vi "Measure Pulsed MinMax Mode.vi"(0 "Current level (A)":dbl=1e-06 format="%_4e", 1 "Current Source Reference In":string="6221", 2 "Voltage Source Reference In":refnum<visa-resource-name>="GPIB0::7::INSTR", 5 "Current Source Range":dbl=1e-05 step=1.0 format="%.4e", 7 "Current Pulse Frequency":dbl=2.0 format="%.4f", 9 "Current Source Compliance (V)":dbl=10.0 min=0.1 max=105.0 step=1.0 format="%.2e", 11 "Averaging time (s)":dbl=20.0, 12 "Voltmeter Wait (ms)":u32=900, 13 "Voltage Buffer Size":i32=60, 14 "Voltmeter Integration (NPLC)":dbl=1.0) -> (4 "Current Source Reference Out":string="6221", 6 "Voltmeter Reference Out":refnum<visa-resource-name>="GPIB0::7::INSTR", 8 "Resistance":dbl=1.1159355882352944, 10 "Error Out Current Source":errorcluster, 15 "Error Out Voltmeter":errorcluster)   [LabVIEW 2020]
uses:
  <vilib>/Analysis/baseanly.llb/Mean (DBL).vi
  <instrlib>/Keithley 2182/Keithley 2182.lvlib
  <vilib>/Analysis/NI_AALBase.lvlib
panel:
  out "i":i32=17
  out "Max-Min (V)":dbl=2.13487e-06
  out "Waveform Chart":dbl(graph)=1.0674350000000001
  in  "Current Pulse Offset":dbl format="%.4e"
  in  "phase mark channel":i32(ring)=1003 items=["TLINK 1"=1001, "TLINK 2"=1002, "TLINK 3"=1003, "TLINK 4"=1004, "None"=-1]
  in  "duty cycle":dbl=50.0 min=0.0 max=100.0 step=10.0 format="%.4f"
  in  "phase mark degrees":dbl=180.0 min=-180.0 max=180.0 step=15.0 format="%.4f"
  in  "Waveform":i32(ring)=2 items=["Sine"=1, "Square"=2, "Triangle"=3, "Ramp Up"=4, "Ramp Down"=5, "DC"=6]
  in  "Error In Voltage source":errorcluster
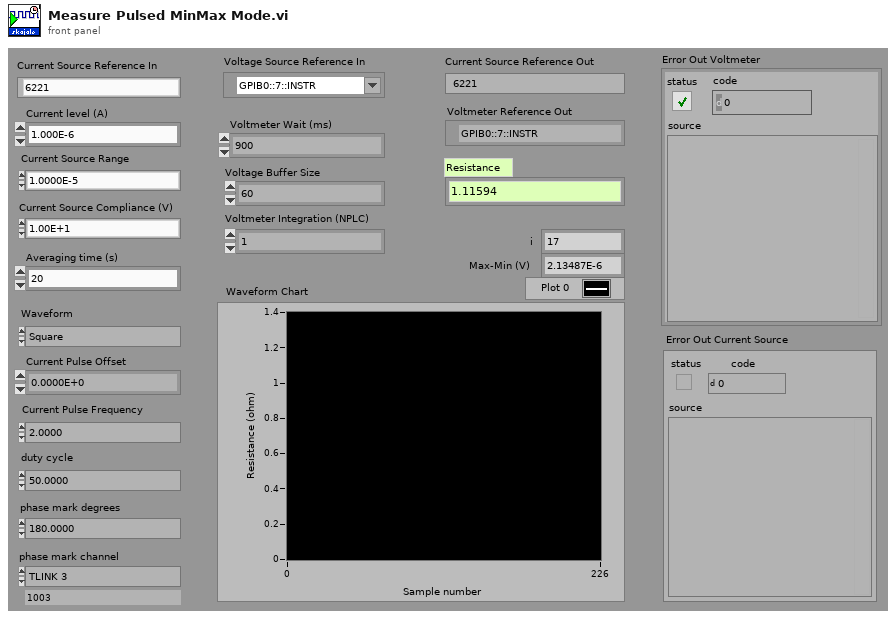
[diagram p1: front panel]
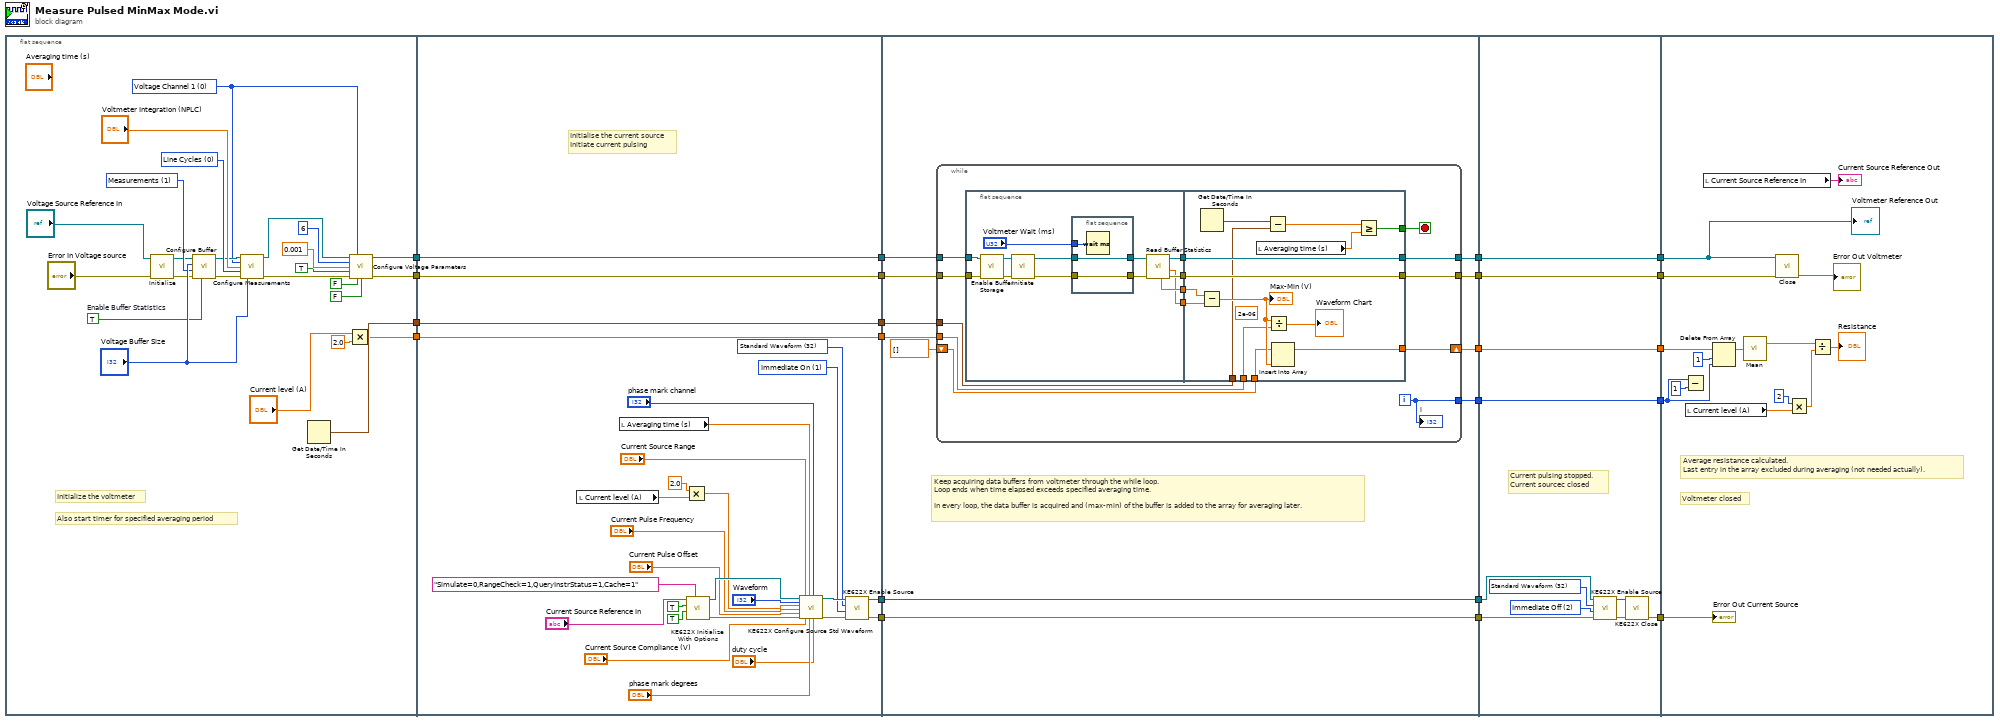
[diagram p0: block diagram]
diagram:
  n1 = flat-sequence {
    tunnel: [w46] -> w20
    tunnel: [w24] -> w5
    tunnel: [w22] -> w3
    tunnel: [w43] -> w1
    tunnel: [w74] -> w21
    tunnel: w20 -> [w74]
    tunnel: [w54] -> w13
    tunnel: [w53] -> w11
    tunnel: [w49] -> w6
    tunnel: w5 -> [w49]
    tunnel: [w48] -> w4
    tunnel: w3 -> [w48]
    tunnel: [w47] -> w2
    tunnel: w1 -> [w47]
    tunnel: w21 -> [w84]
    tunnel: [w83] -> w18
    tunnel: [w82] -> w16
    tunnel: [w81] -> w14
    tunnel: w13 -> [w81]
    tunnel: [w80] -> w12
    tunnel: w11 -> [w80]
    tunnel: [w79] -> w9
    tunnel: [w78] -> w7
    tunnel: w6 -> [w77]
    tunnel: w4 -> [w76]
    tunnel: w2 -> [w75]
    tunnel: [w136] -> w19
    tunnel: w18 -> [w136]
    tunnel: [w135] -> w17
    tunnel: w16 -> [w135]
    tunnel: [w134] -> w15
    tunnel: w14 -> [w133]
    tunnel: w12 -> [w132]
    tunnel: [w131] -> w10
    tunnel: w9 -> [w131]
    tunnel: [w130] -> w8
    tunnel: w7 -> [w130]
    tunnel: w19 -> [w155]
    tunnel: w17 -> [w153]
    tunnel: w15 -> [w145]
    tunnel: w10 -> [w143]
    tunnel: w8 -> [w142]
    frame #0 {
      w26 = 0 items=["Voltage Channel 1", "Voltage Channel 2", "Temperature Channel 1", "Temperature Channel 2"] ("Measurement (0: Voltage Channel 1)")
      w41 = 0 items=["Line Cycles", "Seconds"] ("Integration Rate Units (0: Line Cycles)")
      w37 = 1 items=["None", "Measurements", "Math Calculation"] ("Buffer Source (0: None)")
      w34 = TRUE  # Enable Buffer Statistics
      # "Also start timer for specified averaging period"
      # "Initialize the voltmeter"
      n2 = call <instrlib>:"Initialize.vi"("error in (no error)"="Error In Voltage source", "VISA resource name"="Voltage Source Reference In") -> ("error out"=w36:errorcluster, "VISA resource name out"=w35:refnum<visa-resource-name>)  [unwired: 8 in]
      n3 = call <instrlib>:"Configure Buffer.vi"("Enable Buffer Statistics (0: Disable)"=w34, "error in (no error)"=w36, "Buffer Source (0: None)"=w37, "Buffer Size (2)"="Voltage Buffer Size", "VISA resource name"=w35) -> ("error out"=w40:errorcluster, "VISA resource name out"=w39:refnum<visa-resource-name>)  [unwired: 5 in]
      n4 = call <instrlib>:"Configure Measurements.vi"("VISA resource name"=w39, "Measurement (0: Voltage Channel 1)"=w26, "Integration Rate (5)"="Voltmeter Integration (NPLC)", "Integration Rate Units (0: Line Cycles)"=w41, "error in (no error)"=w40, "Sample Count (1)"="Voltage Buffer Size") -> ("VISA resource name out"=w33:refnum<visa-resource-name>, "error out"=w32:errorcluster)  [unwired: 8 in]
      n5 = Get Date/Time In Seconds() -> (seconds since 1Jan1904=w46:timestamp)
      n6 = Multiply(x="Current level (A)", y=2.0) -> (x*y=w43:dbl)
      n7 = call <instrlib>:"Configure Voltage Parameters.vi"("VISA resource name"=w33, "Measurement (1: Voltage Channel 1)"=w26, "Voltage Resolution (8)"=6, "Range Value (12)"=0.001, "Autorange (T: Enable)"=TRUE, "error in (no error)"=w32, "Enable Ratio (F: Disable)"=FALSE, "Enable Delta (F: Disable)"=FALSE) -> ("VISA resource name out"=w24:refnum<visa-resource-name>, "error out"=w22:errorcluster)  [unwired: 6 in]
    }
    frame #1 {
      w64 = 1 items=["Immediate On"=1, "Immediate Off"=2, "Immediate Standby"=4, "Auto Sync Enabled"=65536, "Auto Sync Disabled"=131072, "Abort On Compliance"=0] ("output action")
      w65 = 32 items=["Bias"=1, "Custom"=8, "DC"=2, "Sweep"=4, "Pulse Gen"=16, "Standard Waveform"=32, "Arbitrary Waveform"=64] ("generator")
      # "Initialise the current source\nInitiate current pulsing"
      n8 = local read "Current level (A)"() -> (w52:dbl)
      n9 = local read "Averaging time (s)"() -> (w55:dbl)
      n10 = Multiply(x=2.0, y=w52) -> (x*y=w51:dbl)
      n11 = call <instrlib>:"KE622X Initialize With Options.vi"("option string"="Simulate=0,RangeCheck=1,QueryInstrStatus=1,Cache=1", "reset device"=TRUE, "id query"=TRUE, "resource name"="Current Source Reference In") -> ("error out"=w66:errorcluster, "instrument handle out"=w67:refnum<k15>)  [unwired: 6 in]
      n12 = call <instrlib>:"KE622X Configure Source Std Waveform.vi"("instrument handle"=w67, "waveform"="Waveform", "amplitude"=w51, "frequency"="Current Pulse Frequency", "dc offset"="Current Pulse Offset", "error in (no error)"=w66, "source range"="Current Source Range", "compliance limit voltage"="Current Source Compliance (V)", "duration"=w55, "phase mark degrees"="phase mark degrees", "phase mark channel"="phase mark channel", "duty cycle"="duty cycle") -> ("instrument handle out"=w68:refnum<k15>, "error out"=w69:errorcluster)  [unwired: 6 in]
      n13 = call <instrlib>:"KE622X Enable Source.vi"("error in (no error)"=w69, "output action"=w64, "generator"=w65, "instrument handle"=w68) -> ("error out"=w53:errorcluster, "instrument handle out"=w54:refnum<k15>)  [unwired: 6 in]
    }
    frame #2 {
      # "Keep acquiring data buffers from voltmeter through the while loop.\nLoop ends when time elapsed exceeds specified averaging time.\n\nIn every loop, the data buffer is acquired and (max-min) of the buffer is added to the array for averaging later."
      n14 = while {
        shift-right: [w88] -> w83
        shift-left: dbl[] [] ("array") -> [w89]
        tunnel: w84 -> [w92]
        tunnel: [w99] -> w82
        tunnel: w76 -> [w98]
        tunnel: w77 -> [w97]
        tunnel: [w96] -> w79
        tunnel: [w95] -> w78
        tunnel: w75 -> [w87]
        i -> [w99]
        stop <- w86 stop-if-true
        n15 = flat-sequence {
          tunnel: w98 -> [w107]
          tunnel: w97 -> [w106]
          tunnel: [w103] -> w94
          tunnel: [w102] -> w93
          tunnel: [w101] -> w91
          tunnel: [w100] -> w90
          tunnel: [w128] -> w95
          tunnel: [w129] -> w96
          tunnel: w94 -> [w129]
          tunnel: w93 -> [w128]
          tunnel: w92 -> [w122]
          tunnel: w91 -> [w121]
          tunnel: w90 -> [w120]
          tunnel: w89 -> [w119]
          tunnel: [w118] -> w88
          tunnel: w87 -> [w116]
          tunnel: [w117] -> w86
          frame #0 {
            n16 = call <instrlib>:"Enable Buffer Storage.vi"("error in (no error)"=w107, "VISA resource name"=w106) -> ("error out"=w105:errorcluster, "VISA resource name out"=w104:refnum<visa-resource-name>)  [unwired: 8 in]
            n17 = call <instrlib>:"Initiate.vi"("error in (no error)"=w105, "VISA resource name"=w104) -> ("error out"=w110:errorcluster, "VISA resource name out"=w112:refnum<visa-resource-name>)  [unwired: 8 in]
            n18 = flat-sequence {
              tunnel: w112 -> [w115]
              tunnel: [w115] -> w111
              tunnel: w110 -> [w114]
              tunnel: [w114] -> w109
              tunnel: "Voltmeter Wait (ms)" -> [w113]
              frame #0 {
                n19 = Wait (ms)(milliseconds to wait=w113) -> ()  [unwired: 1 out]
              }
            }
            n20 = call <instrlib>:"Read Buffer Statistics.vi"("error in (no error)"=w109, "VISA resource name"=w111) -> ("error out"=w102:errorcluster, "Minimum"=w100:dbl, "VISA resource name out"=w103:refnum<visa-resource-name>, "Maximum"=w101:dbl)  [unwired: 4 in, 2 out]
          }
          frame #1 {
            (unwired) 2e-06 ("y")
            n21 = Get Date/Time In Seconds() -> (seconds since 1Jan1904=w123:timestamp)
            n22 = Subtract(x=w121, y=w120) -> (x-y=w126:dbl)
            "Max-Min (V)" <- w126
            n23 = local read "Averaging time (s)"() -> (w125:dbl)
            n24 = Subtract(x=w123, y=w122) -> (x-y=w124:dbl)
            n25 = Divide(x=w126, y=w116) -> (x/y=→"Waveform Chart":dbl)
            n26 = Insert Into Array(array=w119, new element=w126) -> (w118:dbl[])  [unwired: 1 in]
            n27 = Greater Or Equal?(x=w124, y=w125) -> (x >= y?=w117:bool)
          }
        }
        "i" <- w99
      }
    }
    frame #3 {
      w139 = 2 items=["Immediate On"=1, "Immediate Off"=2, "Immediate Standby"=4, "Auto Sync Enabled"=65536, "Auto Sync Disabled"=131072, "Abort On Compliance Enabled"=16777216, "Abort On Compliance Disabled"=33554432] ("output action")
      w140 = 32 items=["Bias"=1, "Custom"=8, "DC"=2, "Sweep"=4, "Pulse Gen"=16, "Standard Waveform"=32, "Arbitrary Waveform"=64] ("generator")
      # "Current pulsing stopped.\nCurrent sourcec closed"
      n28 = call <instrlib>:"KE622X Enable Source.vi"("error in (no error)"=w132, "output action"=w139, "generator"=w140, "instrument handle"=w133) -> ("error out"=w137:errorcluster, "instrument handle out"=w138:refnum<k15>)  [unwired: 6 in]
      n29 = call <instrlib>:"KE622X Close.vi"("error in (no error)"=w137, "instrument handle"=w138) -> ("error out"=w134:errorcluster)  [unwired: 9 in]
    }
    frame #4 {
      # "Voltmeter closed"
      # "Average resistance calculated.\nLast entry in the array excluded during averaging (not needed actually)."
      n30 = Subtract(x=w153, y=1) -> ()  [unwired: 1 out]
      n31 = local read "Current level (A)"() -> (w150:dbl)
      n32 = local read "Current Source Reference In"() -> (→"Current Source Reference Out":string)
      n33 = Delete From Array(array=w155, length=1, index=w153) -> (array with subset deleted=w147:dbl[])  [unwired: 1 out]
      n34 = call-poly <vilib>:"Mean.vi"("X"=w147) -> ("mean"=w146:dbl)  [unwired: 1 out]
      n35 = call <instrlib>:"Close.vi"("error in (no error)"=w142, "VISA resource name"=w143) -> ("error out"=→"Error Out Voltmeter":errorcluster)  [unwired: 9 in]
      n36 = Multiply(x=2 ("value"), y=w150) -> (x*y=w149:dbl)
      n37 = Divide(x=w146, y=w149) -> (x/y=→"Resistance":dbl)
      "Error Out Current Source" <- w145
      "Voltmeter Reference Out" <- w143
    }
  }
